vi "Load Cfg.vi"(8 "error in (no error)":errorcluster, 11 "Socket in":refnum<class "Socket.lvclass">) -> (0 "error out":errorcluster, 3 "Socket out":refnum<class "Socket.lvclass">)   [LabVIEW 2018, in "Socket.lvclass"]
uses:
  Socket.lvclass
  Socket.lvclass/Socket.ctl
  State Machine/CM_State Machine.lvclass/CM_State Machine.ctl
  <vilib>/Utility/config.llb/Read Key (String).vi
  <vilib>/Utility/config.llb/Read Key (Boolean).vi
  <vilib>/Utility/config.llb/Read Key (U32).vi
  <vilib>/Utility/config.llb/NI_LVConfig.lvlib
  State Machine/CM_State Machine.lvclass
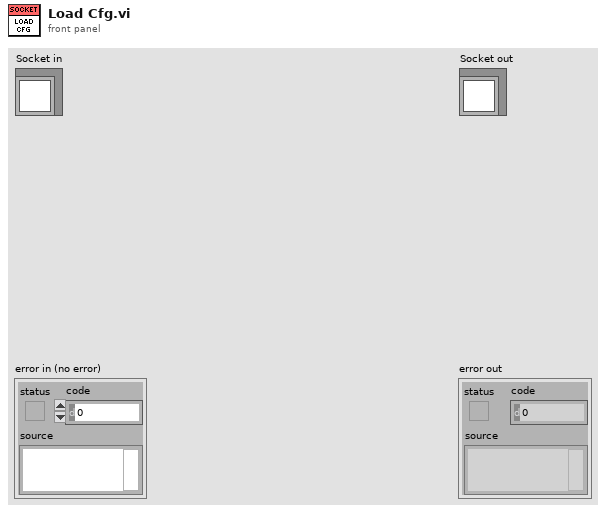
[diagram p1: front panel]
types:
  T1 = typedef "NI_LVConfig.lvlib/Config Data RefNum.ctl" = refnum<k1>
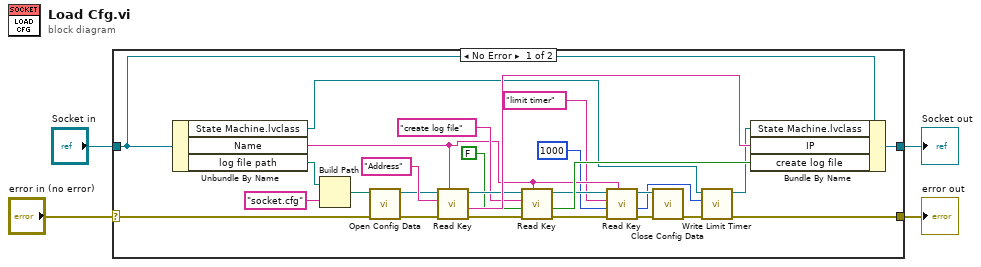
[diagram p0: block diagram]
diagram:
  n1 = case shown="No Error" "error in (no error)" {
    selector: "error in (no error)" -> [w26 w33]
    tunnel: [w15 w33] -> w3
    tunnel: [w24 w32] -> w1
    tunnel: "Socket in" -> [w6 w32]
    frame No Error {
      n2 = Unbundle By Name(w6) -> ("State Machine.lvclass"=w18:refnum<class "CM_State Machine.lvclass">, "Name"=w9:string, "log file path"=w5:path)
      n3 = Build Path(base path=w5, name or relative path="socket.cfg") -> (appended path=w31:path)
      n4 = call <vilib>:"Open Config Data.vi"("error in (no error)"=w26, "configuration file path"=w31) -> ("error out"=w27:errorcluster, "refnum"=w28:T1)  [unwired: 7 in, 1 out]
      n5 = call-poly <vilib>:"Read Key.vi"("section"=w9, "error in (no error)"=w27, "key"="Address", "refnum"=w28) -> ("error out"=w23:errorcluster, "value"=w25:string, "refnum out"=w21:T1)  [unwired: 4 in, 1 out]
      n6 = call-poly <vilib>:"Read Key.vi"("section"=w9, "error in (no error)"=w23, "default value"=FALSE, "key"="create log file", "refnum"=w21) -> ("error out"=w11:errorcluster, "value"=w22:bool, "refnum out"=w14:T1)  [unwired: 3 in, 1 out]
      n7 = call-poly <vilib>:"Read Key.vi"("section"=w9, "error in (no error)"=w11, "default value"=u32 1000, "key"="limit timer", "refnum"=w14) -> ("error out"=w12:errorcluster, "value"=w10:u32, "refnum out"=w13:T1)  [unwired: 3 in, 1 out]
      n8 = call <vilib>:"Close Config Data.vi"("error in (no error)"=w12, "refnum"=w13) -> ("error out"=w16:errorcluster)  [unwired: 8 in, 1 out]
      n9 = call "Write Limit Timer.vi"("error in (no error)"=w16, "Limit Timer"=w10, "State Machine in"=w18) -> ("error out"=w15:errorcluster, "State Machine out"=w17:refnum<class "CM_State Machine.lvclass">)  [unwired: 7 in]
      n10 = Bundle By Name(cluster=w6, "State Machine.lvclass"=w17, "IP"=w25, "create log file"=w22) -> (w24:refnum<class "Socket.lvclass">)
    }
    frame Error {
    }
  }
  "error out" <- w3
  "Socket out" <- w1
